vi "PID Advanced (DBL Array).vi"(0 "setpoint":dbl[](array[numeric])=[0.0] format="%.2f", 1 "output range":cluster{"output high":dbl, "output low":dbl}[](array[cluster])=[{"output high"=100.0, "output low"=-100.0}] {"output low" format="%.2f"; "output high" format="%.2f"}, 2 "auto? (T)":bool[](array[boolean])=[TRUE], 3 "manual control":dbl[](array[numeric])=[0.0] format="%.2f", 5 "process variable":dbl[](array[numeric])=[0.0] format="%.2f", 6 "gamma":dbl[](array[numeric])=[0.0] format="%.2f", 7 "setpoint range":T2(array[cluster])=[{"setpoint high"=100.0, "setpoint low"=0.0}] {"setpoint high" format="%.2f"; "setpoint low" format="%.2f"}, 9 "PID gains":T1(array[cluster])=[{"proportional gain (Kc)"=1.0, "integral time (Ti, min)"=0.01, "derivative time (Td, min)"=0.0}] {"derivative time (Td, min)" format="%.3f"; "integral time (Ti, min)" format="%.3f"; "proportional gain (Kc)" format="%.3f"}, 11 "dt (s)":dbl=-1.0 format="%.3f", 12 "reinitialize? (F)":bool, 13 "beta":dbl[](array[numeric])=[1.0] format="%.2f", 14 "linearity":dbl[](array[numeric])=[1.0] format="%.2f") -> (4 "output":dbl[](array[numeric]) format="%.2f", 15 "dt out (s)":dbl format="%.3f")   [LabVIEW 2020, in "NI_PID_pid.lvlib"]
doc: "Implements a PID controller using a PID algorithm with advanced optional features. The advanced PID algorithm includes the features of the algorithm the PID VI uses, as well as manual mode control with bumpless manual-to-automatic transitions, nonlinear integral action, two degree-of-freedom control, and error-squared control. Use the DBL instance of this VI to implement a single control loop. Use the DBL Array instance to implement parallel multi-loop control."
uses:
  NI_PID_pid.lvlib
  PID Resize 1D Array.vi
  PID Get Advanced Error (DBL).vi
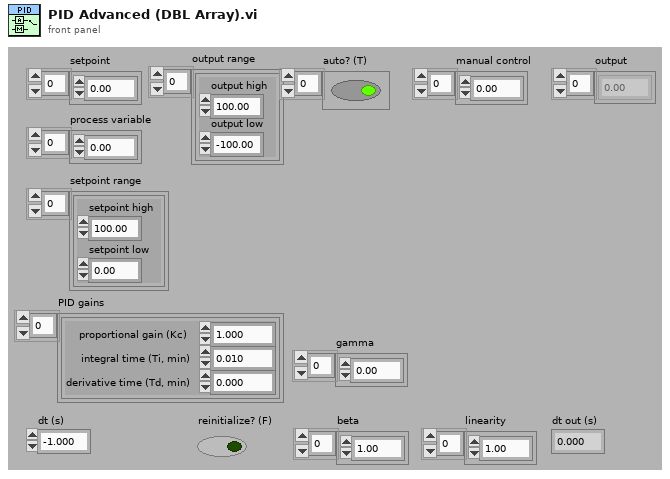
[diagram p1: front panel]
types:
  T1 = cluster{"proportional gain (Kc)":dbl, "integral time (Ti, min)":dbl, "derivative time (Td, min)":dbl}[]
  T2 = cluster{"setpoint high":dbl, "setpoint low":dbl}[]
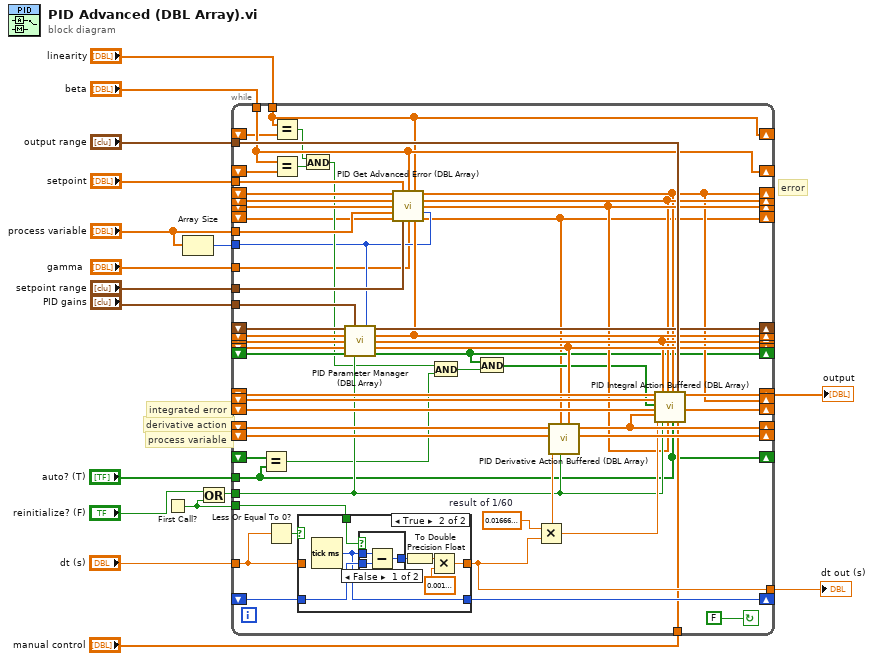
[diagram p0: block diagram]
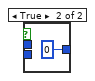
[diagram p3: hidden frame]
diagram:
  # "integrated error"
  # "error"
  # "process variable"
  # "derivative action"
  n1 = First Call?() -> (First Call?: T/F=w16:bool)
  n2 = Array Size(array="process variable") -> (size(s)=w9:i32)
  n3 = Or(x="reinitialize? (F)", y=w16) -> (x .or. y?=w17:bool)
  n4 = while {
    tunnel: w17 -> [w45]
    shift-left: _ -> [w61]
    shift-right: [w60] -> _
    shift-right: [w65] -> _
    shift-left: _ -> [w66]
    shift-right: [w73] -> _
    shift-left: _ -> [w67]
    shift-right: [w72] -> w15
    shift-left: _ -> [w70]
    shift-right: [w36] -> _
    shift-left: _ -> [w71]
    shift-right: [w69] -> _
    shift-left: _ -> [w68]
    tunnel: "dt (s)" -> [w57]
    tunnel: [w59] -> w14
    tunnel: "process variable" -> [w38]
    tunnel: "output range" -> [w62]
    tunnel: w16 -> [w56]
    tunnel: "manual control" -> [w55]
    tunnel: "PID gains" -> [w51]
    shift-right: [w50] -> _
    shift-left: _ -> [w53]
    shift-right: [w49] -> _
    shift-left: _ -> [w52]
    shift-right: [w44] -> _
    shift-left: _ -> [w48]
    shift-right: [w47] -> _
    shift-left: _ -> [w46]
    tunnel: w9 -> [w21]
    shift-right: [w28] -> _
    shift-left: _ -> [w54]
    tunnel: "setpoint range" -> [w43]
    tunnel: "linearity" -> [w32]
    shift-right: [w42] -> _
    shift-left: _ -> [w39]
    tunnel: "setpoint" -> [w37]
    tunnel: "beta" -> [w33]
    shift-right: [w40] -> _
    shift-left: _ -> [w41]
    shift-right: [w36] -> _
    shift-left: _ -> [w35]
    tunnel: "auto? (T)" -> [w23]
    shift-right: [w33] -> _
    shift-left: _ -> [w34]
    shift-right: [w32] -> _
    shift-left: _ -> [w31]
    shift-right: [w23] -> _
    shift-left: _ -> [w24]
    shift-right: [w18] -> _
    shift-left: _ -> [w20]
    tunnel: "gamma" -> [w19]
    stop <- FALSE continue-if-true
    w63 = 0.016666666666666666  # result of 1/60
    n5 = Equal?(x=w24, y=w23) -> (x = y?=w22:bool)
    n6 = Less Or Equal To 0?(x=w57) -> (x <= 0?=w58:bool)
    n7 = Equal?(x=w32, y=w31) -> (x = y?=w30:bool)
    n8 = Equal?(x=w33, y=w34) -> (x = y?=w29:bool)
    n9 = case shown="True" w58 {
      tunnel: [w76 w80] -> w59
      tunnel: w61 -> [w75 w79]
      tunnel: [w75 w78] -> w60
      tunnel: w57 -> [w76 _]
      tunnel: w56 -> [_ w77]
      frame False {
      }
      frame True {
        n10 = Tick Count (ms)() -> (millisecond timer value=w78:u32)
        n11 = case shown="False" w77 {
          tunnel: [w86 u32 0] -> w82
          tunnel: w79 -> [w85 _]
          tunnel: w78 -> [w84 _]
          frame False {
            n12 = Subtract(x=w84, y=w85) -> (x-y=w86:u32)
          }
          frame True {
          }
        }
        n13 = To Double Precision Float(number=w82) -> (double precision float=w81:dbl)
        n14 = Multiply(x=w81, y=0.0010000000474974513) -> (x*y=w80:dbl)
      }
    }
    n15 = And(x=w30, y=w29) -> (x .and. y?=w26:bool)
    n16 = call "PID Parameter Manager (DBL Array).vi"("previous PID gains"=w46, "PID gains"=w51, "process variable size"=w21, "previous Kp"=w48, "previous Ki"=w52, "previous Kd"=w53, "previous PID Gains equal ?"=w54, "initialize"=w45) -> ("PID Parameter Out"=w47:T1, "Kp"=w44:dbl[], "Ki"=w49:dbl[], "Kd"=w50:dbl[], "PID Gains equal ?"=w28:bool[])  [unwired: 3 out]
    n17 = call "PID Get Advanced Error (DBL Array).vi"("error buffer"=w35, "setpoint"=w37, "beta"=w33, "linearity"=w32, "error (with beta) buffer"=w41, "non-linear integral buffer"=w39, "process variable"=w38, "process variable size"=w21, "error (with gamma) buffer"=w20, "setpoint range"=w43, "gamma"=w19, "Kp"=w44) -> ("error"=w36:dbl[], "error (with beta)"=w40:dbl[], "non-linear integral"=w42:dbl[], "error (with gamma)"=w18:dbl[])
    n18 = And(x=w26, y=w22) -> (x .and. y?=w25:bool)
    n19 = And(x=w28, y=w25) -> (x .and. y?=w27:bool[])
    n20 = Multiply(x=w63, y=w59) -> (x*y=w64:dbl)
    n21 = call "PID Derivative Action Buffered (DBL Array).vi"("Kd"=w50, "initialize (F)"=w45, "process variable"=w18, "dt (min)"=w64, "previous  process variable"=w67, "previous derivative action"=w66) -> ("process variable buffer"=w73:dbl[], "derivative action"=w65:dbl[])  [unwired: 1 in, 3 out]
    n22 = call "PID Integral Action Buffered (DBL Array).vi"("previous output"=w70, "previous error"=w71, "PID Gains equal?"=w27, "previous integrated error"=w68, "previous derivative action"=w65, "dt (min)"=w64, "Ki"=w49, "initialize (F)"=w45, "proportional action"=w40, "linearity ([1])"=w42, "error"=w36, "auto? (T)"=w23, "output range"=w62, "manual control"=w55) -> ("output"=w72:dbl[], "integrated error out"=w69:dbl[])  [unwired: 1 in, 3 out]
  }
  "dt out (s)" <- w14
  "output" <- w15
